vi "create.ModifyOrderShort.vi"(8 "error in":errorcluster, 10 "ModifyOrderShort.Parameters":T1={"Time Offset"=447000, "Order Id"="ORID0001", "Quantity"=20000, "Price"=1, "Modify Flags"=1}, 11 "ModifyOrderShort in":refnum<class "ModifyOrderShort.lvclass">) -> (0 "error out":errorcluster, 3 "ModifyOrderShort out":refnum<class "ModifyOrderShort.lvclass">)   [LabVIEW 2020, in "ModifyOrderShort.lvclass"]
uses:
  ModifyOrderShort.lvclass
  ModifyOrderShort.Parameters.ctl
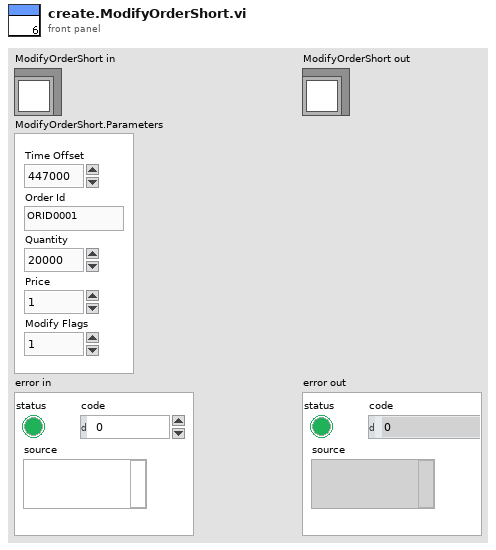
[diagram p1: front panel]
types:
  T1 = typedef "ModifyOrderShort.lvclass/ModifyOrderShort.Parameters.ctl" = cluster{"Time Offset":u32, "Order Id":string, "Quantity":u32, "Price":u16, "Modify Flags":u8}
  T2 = enum16{"Alphanumeric", "Binary", "BinaryLongPrice", "BinaryShortPrice", "BitField", "PrintableAscii", "Value"}
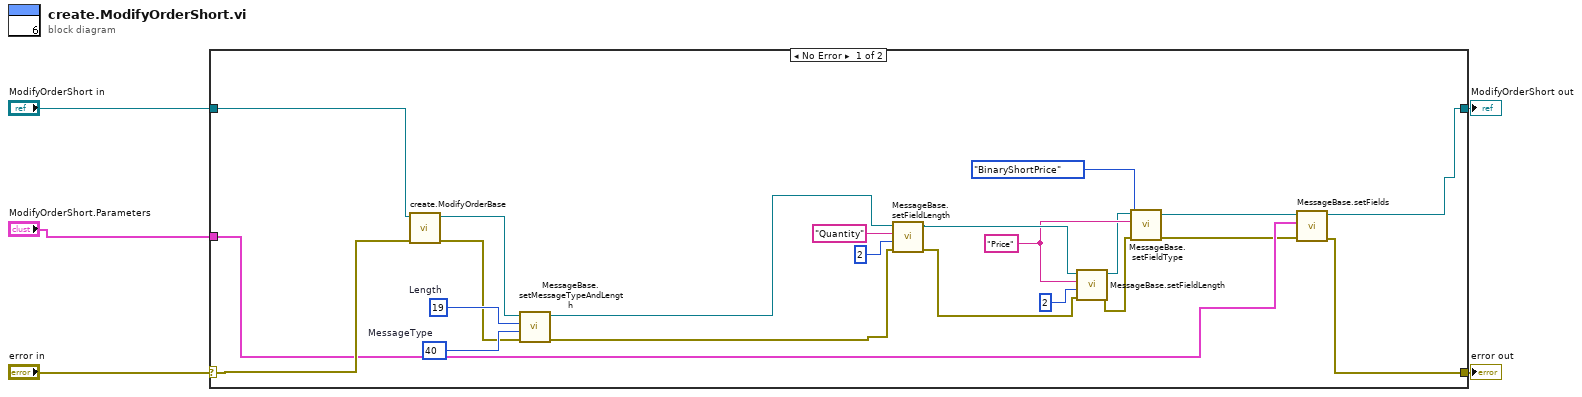
[diagram p0: block diagram]
diagram:
  n1 = case shown="No Error" "error in" {
    selector: "error in" -> [w16 w29]
    tunnel: [w14 w29] -> w4
    tunnel: [w12 w28] -> w2
    tunnel: "ModifyOrderShort in" -> [w13 w28]
    tunnel: "ModifyOrderShort.Parameters" -> [w15 _]
    frame No Error {
      w11 = "Price" ("Field.Name")
      w26 = u8 40  # MessageType
      w27 = u8 19  # Length
      n2 = call-dynamic "create.ModifyOrderBase.vi"("error in (no error)"=w16, "ModifyOrderBase in"=w13) -> ("error out"=w24:errorcluster, "ModifyOrderBase out"=w25:refnum<class "ModifyOrderShort.lvclass">)  [unwired: 8 in]
      n3 = call-dynamic "MessageBase.setMessageTypeAndLength.vi"("error in (no error)"=w24, "MessageType"=w26, "Length"=w27, "MessageBase in"=w25) -> ("error out"=w17:errorcluster, "MessageBase out"=w18:refnum<class "ModifyOrderShort.lvclass">)  [unwired: 6 in]
      n4 = call-dynamic "MessageBase.setFieldLength.vi"("error in (no error)"=w17, "Length"=2, "FIeld.Name"="Quantity" ("Field.Name"), "MessageBase in"=w18) -> ("error out"=w19:errorcluster, "MessageBase out"=w20:refnum<class "ModifyOrderShort.lvclass">)  [unwired: 6 in]
      n5 = call-dynamic "MessageBase.setFieldLength.vi"("error in (no error)"=w19, "Length"=2, "FIeld.Name"=w11, "MessageBase in"=w20) -> ("error out"=w9:errorcluster, "MessageBase out"=w10:refnum<class "ModifyOrderShort.lvclass">)  [unwired: 6 in]
      n6 = call-dynamic "MessageBase.setFieldType.vi"("error in (no error)"=w9, "FieldType"=T2."BinaryShortPrice", "FIeld.Name"=w11, "MessageBase in"=w10) -> ("error out"=w8:errorcluster, "MessageBase out"=w7:refnum<class "ModifyOrderShort.lvclass">)  [unwired: 6 in]
      n7 = call-dynamic "MessageBase.setFields.vi"("error in (no error)"=w8, "Cluster (dup)"=w15, "MessageBase in"=w7) -> ("error out"=w14:errorcluster, "MessageBase out"=w12:refnum<class "ModifyOrderShort.lvclass">)  [unwired: 7 in]
    }
    frame Error {
    }
  }
  "error out" <- w4
  "ModifyOrderShort out" <- w2
